vi "Start Acquiring.vi"(6 "wait for reply (T)":bool=TRUE, 8 "error in (no error)":errorcluster, 11 "Module ID":i32=-1) -> (0 "error out":errorcluster, 1 "timed out?":bool, 2 "Reply Payload":T1)   [LabVIEW 2018, in "LGP5 Acquisition.lvlib"]
doc: "The Start Acquiring request event requests the module to configure the DAQ device and start acquiring.\nThe Acquisition Started broadcast event indicates when the DAQ device has started aquiring.\n_____\nCreated using Delacor QMH Event Scripter 4.2.0.84."
uses:
  LGP5 Acquisition.lvlib
  Start Acquiring (Reply Payload)--cluster.ctl
  Start Acquiring Argument--cluster.ctl
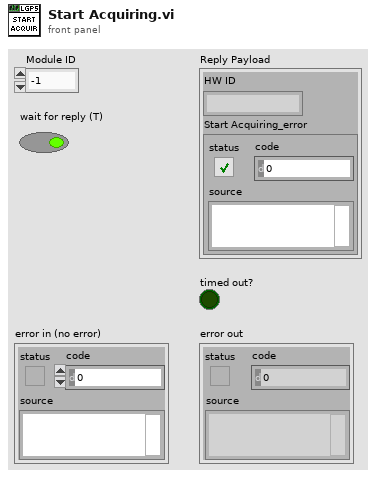
[diagram p1: front panel]
types:
  T1 = typedef "LGP5 Acquisition.lvlib/Start Acquiring (Reply Payload)--cluster.ctl" = cluster{"HW ID":string, "Start Acquiring_error":errorcluster}
  T2 = typedef "LGP5 Acquisition.lvlib/Start Acquiring Argument--cluster.ctl" = cluster{"Module ID":i32, "Wait Notifier":refnum<notifier>, "wait for reply":bool}
  T3 = typedef "LGP5 Acquisition.lvlib/Request Events--cluster.ctl" = cluster{"Stop Module":refnum<user-event>, "Show Panel":refnum<user-event>, "Hide Panel":refnum<user-event>, "Show Diagram":refnum<user-event>, "Get Module Execution Status":refnum<user-event>, "Start Acquiring":refnum<user-event>}
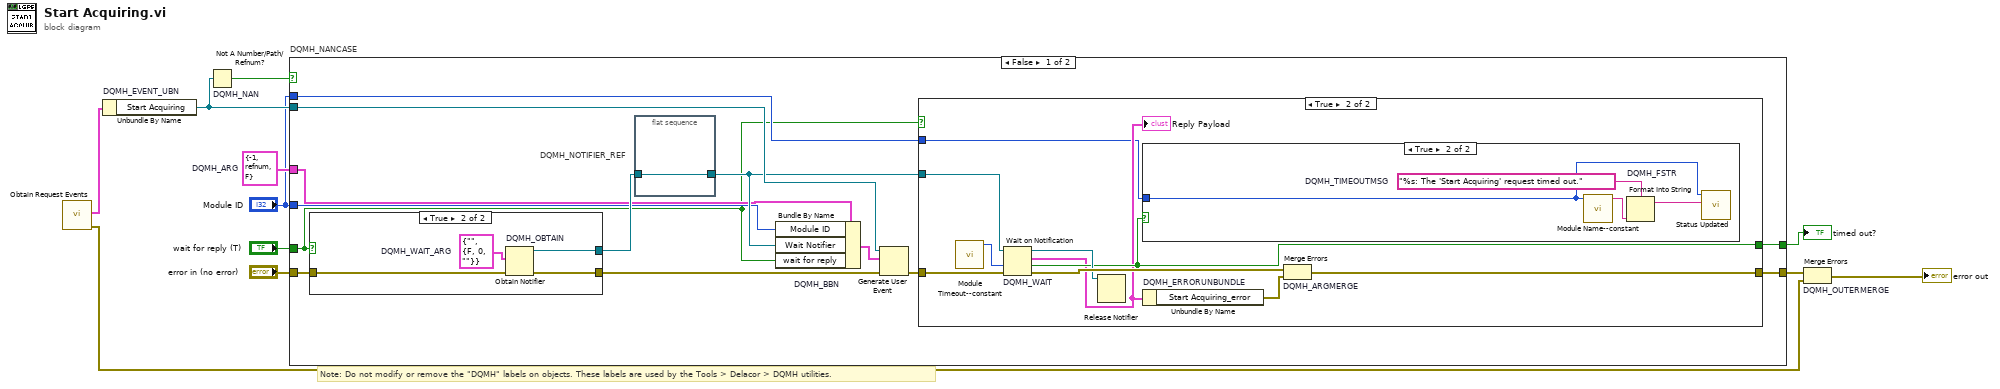
[diagram p0: block diagram]
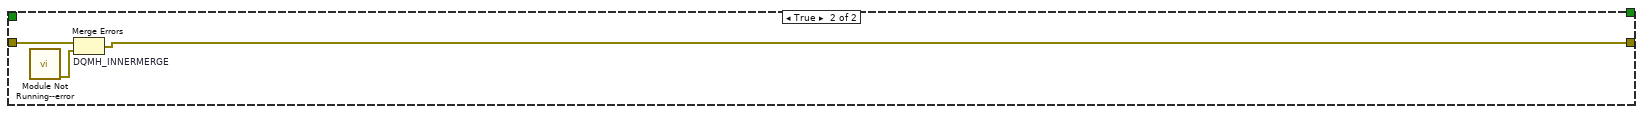
[diagram p5: hidden frame]
diagram:
  w5 = T2 {"Module ID"=-1, "Wait Notifier"=refnum, "wait for reply"=FALSE}  # DQMH_ARG
  # "Note: Do not modify or remove the \"DQMH\" labels on objects. These labels are used by the Tools > Delacor > DQMH utilities."
  n1 = call "Obtain Request Events.vi"() -> ("error out"=w2:errorcluster, "LGP5 Acquisition Request Events"=w1:T3)  [unwired: 10 in]
  n2 = Unbundle By Name "DQMH_EVENT_UBN"(w1) -> ("Start Acquiring"=w9:refnum<user-event>)
  n3 = Not A Number/Path/Refnum? "DQMH_NAN"(number/path/refnum=w9) -> (NaN/Path/Refnum?=w8:bool)
  n4 = case "DQMH_NANCASE" shown="False" w8 {
    tunnel: "error in (no error)" -> [w24 w48]
    tunnel: w9 -> [w22 _]
    tunnel: [w19 w47] -> w6
    tunnel: [w20 _] -> w7
    tunnel: w5 -> [w15 _]
    tunnel: "Module ID" -> [w14 _]
    tunnel: "Module ID" -> [w13 _]
    tunnel: "wait for reply (T)" -> [w12 _]
    frame False {
      n5 = case shown="True" w12 {
        tunnel: w24 -> [w41 w45]
        tunnel: [w41 w44] -> w21
        tunnel: [_ w42] -> w17
        frame False {
        }
        frame True {
          w43 = T1 {"HW ID"="", "Start Acquiring_error"={"status"=FALSE, "code"=0, "source"=""}}  # DQMH_WAIT_ARG
          n6 = Obtain Notifier "DQMH_OBTAIN"(notification data type=w43, error in (no error)=w45) -> (notifier out=w42:refnum<notifier>, error out=w44:errorcluster)  [unwired: 2 in, 1 out]
        }
      }
      n7 = flat-sequence "DQMH_NOTIFIER_REF" {
        tunnel: w17 -> [w25]
        tunnel: [w25] -> w16
        frame #0 {
        }
      }
      n8 = Bundle By Name "DQMH_BBN"(cluster=w15, "Module ID"=w14, "Wait Notifier"=w16, "wait for reply"=w12) -> (w18:T2)
      n9 = Generate User Event(user event=w22, event data cluster=w18, error in=w21) -> (error out=w23:errorcluster)  [unwired: 1 in, 1 out]
      n10 = case shown="True" w12 {
        tunnel: w23 -> [w26 w36]
        tunnel: w16 -> [_ w34]
        tunnel: [_ w32] -> w20
        tunnel: [w26 w31] -> w19
        tunnel: w13 -> [_ w27]
        frame False {
        }
        frame True {
          n11 = call "Module Timeout--constant.vi"() -> ("Module Timeout"=w28:i32)  [unwired: 11 in]
          n12 = Wait on Notification "DQMH_WAIT"(notifier=w34, timeout in ms (-1)=w28, error in (no error)=w36) -> (notifier out=w33:refnum<notifier>, notification=w29:T1, timed out?=w32:bool, error out=w35:errorcluster)  [unwired: 1 in]
          "Reply Payload" <- w29
          n13 = Release Notifier(notifier=w33) -> ()  [unwired: 2 in, 3 out]
          n14 = case shown="True" w32 {
            tunnel: w27 -> [_ w37]
            frame False {
            }
            frame True {
              w40 = "%s: The 'Start Acquiring' request timed out."  # DQMH_TIMEOUTMSG
              n15 = call "Module Name--constant.vi"("Module ID"=w37) -> ("Module Name"=w39:string)  [unwired: 10 in]
              n16 = Format Into String "DQMH_FSTR"(format string=w40, w39) -> (resulting string=w38:string)  [unwired: 2 in, 1 out]
              n17 = call "Status Updated.vi"("Status"=w38, "Module ID"=w37) -> ()  [unwired: 9 in, 1 out]
            }
          }
          n18 = Unbundle By Name "DQMH_ERRORUNBUNDLE"(w29) -> ("Start Acquiring_error"=w30:errorcluster)
          n19 = Merge Errors "DQMH_ARGMERGE"(w35, w30) -> (w31:errorcluster)
        }
      }
    }
    frame True {
      n20 = call "Module Not Running--error.vi"() -> ("error out"=w46:errorcluster)  [unwired: 11 in]
      n21 = Merge Errors "DQMH_INNERMERGE"(w48, w46) -> (w47:errorcluster)
    }
  }
  "timed out?" <- w7
  n22 = Merge Errors "DQMH_OUTERMERGE"(w6, w2) -> (→"error out":errorcluster)
